vi "Resample VR Data.vi"(7 "Memory Size":i32=32768, 11 "Data In":dbl[](array[numeric])) -> (3 "Resampled Data":dbl[](array[numeric]))   [LabVIEW 2013, in "Data Replay File.lvlib"]
uses:
  Data Replay File.lvlib
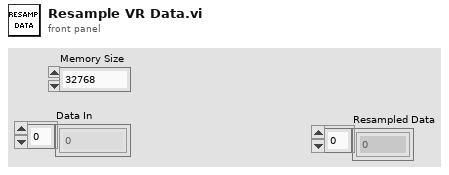
[diagram p1: front panel]
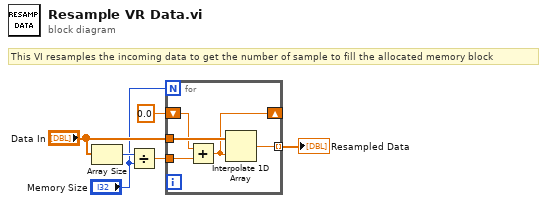
[diagram p0: block diagram]
diagram:
  # "This VI resamples the incoming data to get the number of sample to fill the allocated memory block"
  n1 = Array Size(array="Data In") -> (size(s)=w4:i32)
  n2 = Divide(x=w4, y="Memory Size") -> (x/y=w1:dbl)
  n3 = for {
    N: "Memory Size" -> [_]
    tunnel: "Data In" -> [w11]
    tunnel: [w10] -> w6 mode=indexing
    shift-right: [w7] -> _
    shift-left: 0.0 -> [w9]
    tunnel: w1 -> [w8]
    n4 = Add(x=w9, y=w8) -> (x+y=w7:dbl)
    n5 = Interpolate 1D Array(1:w7, 2:w11) -> (0:w10:dbl)
  }
  "Resampled Data" <- w6
